vi "Teleop.vi"(10 "Match Info":T1={"Autonomous Elapsed Seconds"=0.0, "TeleOp Elapsed Seconds"=0.0, "Disabled Elapsed Seconds"=0.0, "Visited Autonomous"=FALSE, "Visited TeleOp"=FALSE, "Visited Disabled"=FALSE, "Autonomous Settings"={"Autonomous Style"=enum."Independent", "VI Refnum"=refnum}}, 11 "Call Context":T2) -> ()   [LabVIEW 2015]
doc: "This VI is called for each enabled TeleOp packet received from the DS. It is typically used to read from joysticks and other inputs and update I/O or setpoints for timed control loops. It should complete and return within 20 milliseconds or risk missing DS packets."
uses:
  <vilib>/Rock Robotics/WPI/DriverStation/WPI_DriverStationDerivedRobotMode.ctl
  <vilib>/Rock Robotics/WPI/DriverStation/WPI_DriverStationMatch Info.ctl
  Shooter/Implementation/Shooter Operations.ctl
  Support Code/Team900-VIs/Logitech/F510/F510-X.vi
  Shooter/Implementation/Shooter Published Globals.vi
  Drive/Implementation/Drive Operations.ctl
  Drive/Implementation/Drive Published Globals.vi
panel:
  in  "Angle":dbl=90.0 format="%#_13g"
  in  "Y":i32=40
  in  "X":i32=5
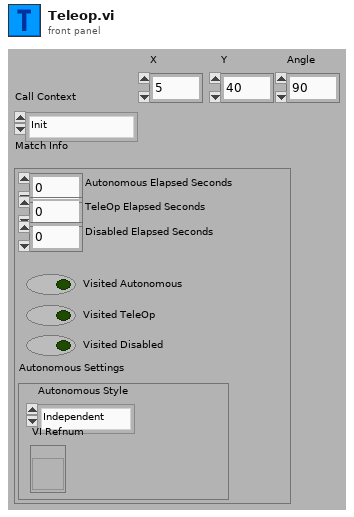
[diagram p1: front panel]
types:
  T1 = typedef "WPI_DriverStationMatch Info.ctl" = cluster{"Autonomous Elapsed Seconds":dbl, "TeleOp Elapsed Seconds":dbl, "Disabled Elapsed Seconds":dbl, "Visited Autonomous":bool, "Visited TeleOp":bool, "Visited Disabled":bool, "Autonomous Settings":cluster{"Autonomous Style":enum16{"Iterative", "Independent"}, "VI Refnum":refnum<vi>}}
  T2 = typedef "WPI_DriverStationDerivedRobotMode.ctl" = enum16{"Init", "Execute", "Stop"}
  T3 = typedef "Shooter Operations.ctl" = enum16{"Reserve", "Read Current", "Immediate", "Fire", "Aim"}
  T4 = typedef "Shooter Setpoints.ctl" = cluster{"Operation":T3, "Setpoint":dbl, "Duration":dbl}
  T5 = cluster{"A":bool, "B":bool, "X":bool, "Y":bool, "LB":bool, "RB":bool, "Back":bool, "Start":bool, "LC":bool, "RC":bool, "LT":bool, "RT":bool}
  T6 = typedef "Drive Operations.ctl" = enum16{"Reserve", "Read Current", "Immediate", "Turn to Angle", "Pick Up Ball", "Drive Straight", "Drive to Target (arc)"}
  T7 = typedef "Drive Setpoints.ctl" = cluster{"Operation":T6, "Left Setpoint":dbl, "Right Setpoint":dbl, "Duration":dbl, "Position":cluster{"X":dbl, "Y":dbl, "Angle":dbl, "Distance":dbl}, "Straight Setpoint":dbl}
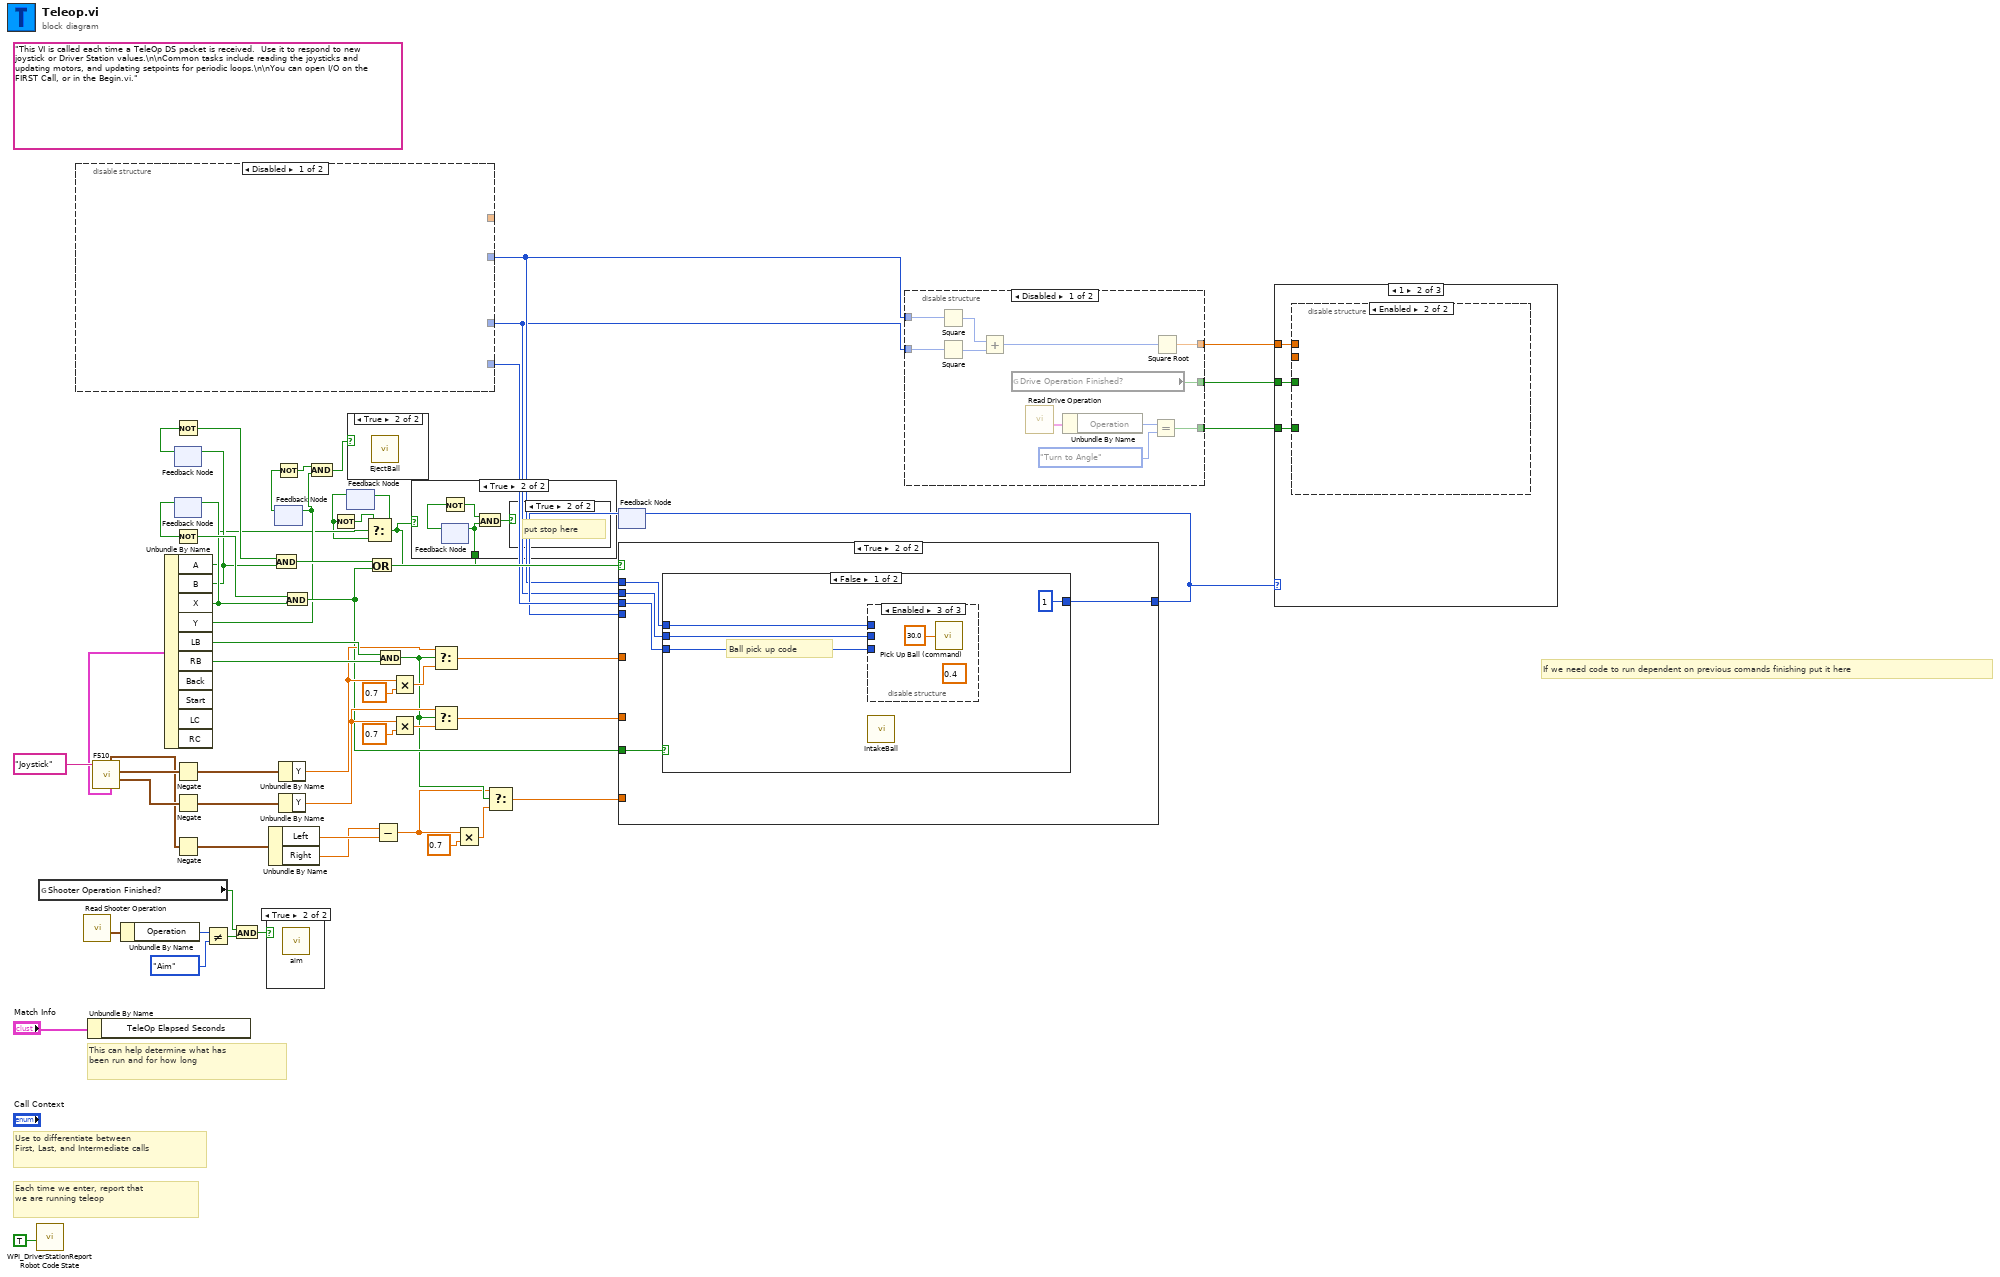
[diagram p0: block diagram]
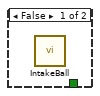
[diagram p2: hidden frame]
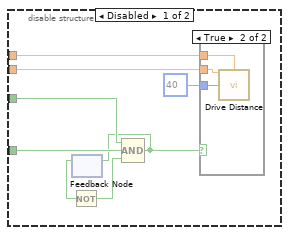
[diagram p8: hidden frame]
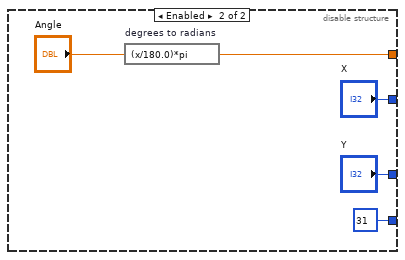
[diagram p11: hidden frame]
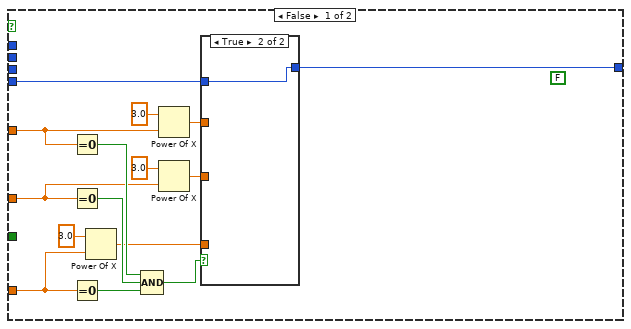
[diagram p12: hidden frame]
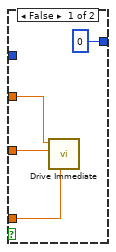
[diagram p13: hidden frame]
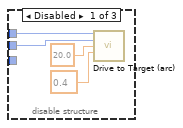
[diagram p14: hidden frame]
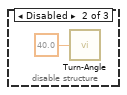
[diagram p15: hidden frame]
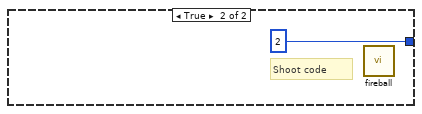
[diagram p16: hidden frame]
diagram:
  (unwired) "This VI is called each time a TeleOp DS packet is received.  Use it to respond to new joystick or Driver Station values.\n\nCommon tasks include reading the joysticks and updating motors, and updating setpoints for periodic loops.\n\nYou can open I/O on the FIRST Call, or in the Begin.vi."
  # "If we need code to run dependent on previous comands finishing put it here"
  # "Each time we enter, report that\nwe are running teleop"
  # "Use to differentiate between\nFirst, Last, and Intermediate calls"
  # "This can help determine what has\nbeen run and for how long"
  n1 = call <vilib>:"WPI_DriverStationReport Robot Code State.vi"("TeleOp"=TRUE ("Autonomous")) -> ()  [unwired: 10 in, 1 out]
  n2 = global read "Shooter Published Globals.vi" "Shooter Operation Finished?"() -> (w9:bool)
  n3 = disable-structure shown="Disabled" {
    disable-tunnel: [_ 31] -> w32
    disable-tunnel: [_ "Y"] -> w20
    disable-tunnel: [_ "X"] -> w21
    disable-tunnel: [_ w59] -> _
    frame Disabled {
    }
    frame Enabled {
      n4 = expression code="(x/180.0)*pi" "degrees to radians"("Angle") -> (w59:dbl)
    }
  }
  n5 = call "Read Shooter Operation.vi"() -> ("SubSystem Data"=w14:T4)  [unwired: 10 in, 1 out]
  n6 = Unbundle By Name("Match Info") -> ()  [unwired: 1 out]
  n7 = call-poly "F510.vi"("refnum name"="Joystick") -> ("Right Stick"=w54:cluster{"X":dbl, "Y":dbl}, "Left Stick"=w55:cluster{"X":dbl, "Y":dbl}, "Buttons"=w53:T5, "Triggers"=w52:cluster{"Left":dbl, "Right":dbl})  [unwired: 4 in, 3 out]
  n8 = Unbundle By Name(w14) -> ("Operation"=w13:T3)
  n9 = Unbundle By Name(w53) -> ("A"=w4:bool, "B"=w37:bool, "X"=w44:bool, "Y"=w6:bool, "LB"=w50:bool, "RB"=w51:bool)  [unwired: 4 out]
  n10 = feedback #1() -> (w36:bool)  [unwired: 1 in]
  n11 = Not(x=w36) -> (.not. x?=w38:bool)
  n12 = feedback-in #1(w37) -> ()
  n13 = feedback #2() -> (w41:bool)  [unwired: 1 in]
  n14 = feedback-in #2(w44) -> ()
  n15 = Not(x=w41) -> (.not. x?=w45:bool)
  n16 = Negate(x=w55) -> (-x=w16:cluster{"X":dbl, "Y":dbl})
  n17 = Negate(x=w54) -> (-x=w15:cluster{"X":dbl, "Y":dbl})
  n18 = Negate(x=w52) -> (-x=w17:cluster{"Left":dbl, "Right":dbl})
  n19 = Not Equal?(x=w13, y=Shooter_Operations."Aim") -> (x != y?=w11:bool)
  n20 = And(x=w9, y=w11) -> (x .and. y?=w10:bool)
  n21 = case shown="True" w10 {
    frame False {
    }
    frame True {
      n22 = call "aim.vi"() -> ()  [unwired: 11 in, 1 out]
    }
  }
  n23 = Unbundle By Name(w17) -> ("Left"=w27:dbl, "Right"=w26:dbl)
  n24 = And(x=w38, y=w37) -> (x .and. y?=w35:bool)
  n25 = feedback #3() -> (w8:bool)  [unwired: 1 in]
  n26 = Not(x=w8) -> (.not. x?=w7:bool)
  n27 = feedback-in #3(w6) -> ()
  n28 = Unbundle By Name(w16) -> ("Y"=w42:dbl)
  n29 = Unbundle By Name(w15) -> ("Y"=w43:dbl)
  n30 = And(x=w45, y=w44) -> (x .and. y?=w33:bool)
  n31 = And(x=w7, y=w6) -> (x .and. y?=w5:bool)
  n32 = feedback #4() -> (w2:bool)  [unwired: 1 in]
  n33 = Not(x=w2) -> (.not. x?=w3:bool)
  n34 = case shown="True" w5 {
    frame False {
    }
    frame True {
      n35 = call "EjectBall.vi"() -> ()  [unwired: 11 in, 1 out]
    }
  }
  n36 = Select(t=w3, s=w4, f=w2) -> (s? t:f=w1:bool)
  n37 = feedback-in #4(w1) -> ()
  n38 = Or(x=w35, y=w33) -> (x .or. y?=w34:bool)
  n39 = Subtract(x=w26, y=w27) -> (x-y=w25:dbl)
  n40 = And(x=w50, y=w51) -> (x .and. y?=w31:bool)
  n41 = Multiply(x=w42, y=0.7) -> (x*y=w47:dbl)
  n42 = Multiply(x=w43, y=0.7) -> (x*y=w49:dbl)
  n43 = case shown="True" w1 {
    tunnel: w1 -> [_ w65]
    frame False {
      n44 = call "IntakeBall.vi"() -> ()  [unwired: 11 in, 1 out]
    }
    frame True {
      n45 = feedback #5() -> (w67:bool)  [unwired: 1 in]
      n46 = Not(x=w67) -> (.not. x?=w66:bool)
      n47 = feedback-in #5(w65) -> ()
      n48 = And(x=w66, y=w65) -> (x .and. y?=w64:bool)
      n49 = case shown="True" w64 {
        frame False {
        }
        frame True {
          # "put stop here"
        }
      }
    }
  }
  n50 = Select(t=w42, s=w31, f=w47) -> (s? t:f=w40:dbl)
  n51 = Select(t=w43, s=w31, f=w49) -> (s? t:f=w39:dbl)
  n52 = Multiply(x=w25, y=0.7) -> (x*y=w29:dbl)
  n53 = Select(t=w25, s=w31, f=w29) -> (s? t:f=w28:dbl)
  n54 = feedback #6() -> (w23:i32)  [unwired: 1 in]
  n55 = case shown="True" w34 {
    tunnel: w40 -> [w78 _]
    tunnel: w39 -> [w73 _]
    tunnel: w33 -> [_ w92]
    tunnel: w32 -> [_ w91]
    tunnel: w20 -> [_ w90]
    tunnel: w21 -> [_ w89]
    tunnel: w28 -> [w71 _]
    tunnel: [w68 w88] -> w24
    tunnel: w23 -> [w69 _]
    frame False {
      (unwired) FALSE
      n56 = Equal To 0?(x=w78) -> (x = 0?=w81:bool)
      n57 = Equal To 0?(x=w73) -> (x = 0?=w82:bool)
      n58 = Equal To 0?(x=w71) -> (x = 0?=w79:bool)
      n59 = Power Of X(1:w71, 2:3.0 ("y")) -> (0:w70:dbl)
      n60 = Compound Arithmetic op=AND(w81, w82, w79) -> (w80:bool)
      n61 = Power Of X(1:w78, 2:3.0 ("y")) -> (0:w77:dbl)
      n62 = Power Of X(1:w73, 2:3.0 ("y")) -> (0:w74:dbl)
      n63 = case shown="True" w80 {
        tunnel: w77 -> [w86 _]
        tunnel: w74 -> [w85 _]
        tunnel: w70 -> [w84 _]
        tunnel: w69 -> [_ w87]
        tunnel: [0 w87] -> w68
        frame False {
          n64 = call "Drive Immediate.vi"("Straight Setpoint"=w84, "Right Setpoint"=w85, "Left Setpoint"=w86) -> ()  [unwired: 8 in, 1 out]
        }
        frame True {
        }
      }
    }
    frame True {
      n65 = case shown="False" w92 {
        tunnel: w91 -> [w96 _]
        tunnel: w90 -> [w94 _]
        tunnel: w89 -> [w95 _]
        tunnel: [1 2] -> w88
        frame False {
          # "Ball pick up code"
          n66 = disable-structure shown="Enabled" {
            disable-tunnel: w96 -> [_ _ _]
            disable-tunnel: w94 -> [w98 _ _]
            disable-tunnel: w95 -> [w100 _ _]
            frame Disabled {
              n67 = call "Drive to Target (arc).vi"("X"=w100, "Y"=w98, "Max time"=20.0, "Speed Setpoint (-1 to 1"=0.4) -> ()  [unwired: 10 in, 2 out]
            }
            frame Disabled {
              n68 = call "Turn-Angle.vi"("Max time"=40.0) -> ("Angle"=w102:dbl)  [unwired: 12 in, 2 out]
            }
            frame Enabled {
              (unwired) 0.4
              n69 = call "Pick Up Ball (command).vi"("Max time"=30.0) -> ()  [unwired: 13 in, 2 out]
            }
          }
          n70 = call "IntakeBall.vi"() -> ()  [unwired: 11 in, 1 out]
        }
        frame True {
          # "Shoot code"
          n71 = call "fireball.vi"() -> ()  [unwired: 11 in, 1 out]
        }
      }
    }
  }
  n72 = feedback-in #6(w24) -> ()
  n73 = disable-structure shown="Disabled" {
    disable-tunnel: [w115 _] -> w22
    disable-tunnel: w21 -> [w111 _]
    disable-tunnel: w20 -> [w110 _]
    disable-tunnel: [w109 _] -> w19
    disable-tunnel: [w105 _] -> w18
    frame Disabled {
      n74 = Square(x=w111) -> (x^2=w114:i32)
      n75 = Square(x=w110) -> (x^2=w112:i32)
      n76 = Add(x=w114, y=w112) -> (x+y=w113:i32)
      n77 = global read "Drive Published Globals.vi" "Drive Operation Finished?"() -> (w115:bool)
      n78 = call "Read Drive Operation.vi"() -> ("SubSystem Data"=w108:T7)  [unwired: 10 in, 1 out]
      n79 = Unbundle By Name(w108) -> ("Operation"=w107:T6)
      n80 = Equal?(x=w107, y=Drive_Operations."Turn to Angle") -> (x = y?=w105:bool)
      n81 = Square Root(x=w113) -> (sqrt(x)=w109:dbl)
    }
    frame Enabled {
    }
  }
  n82 = case shown="1" w24 {
    tunnel: w22 -> [_ w117 _]
    tunnel: w19 -> [_ w118 _]
    tunnel: w18 -> [_ w116 _]
    frame 0, Default {
    }
    frame 1 {
      n83 = disable-structure shown="Enabled" {
        disable-tunnel: _ -> [w126 _]
        disable-tunnel: w118 -> [w125 _]
        disable-tunnel: w117 -> [w124 _]
        disable-tunnel: w116 -> [w123 _]
        frame Disabled {
          n84 = feedback #7() -> (w121:bool)  [unwired: 1 in]
          n85 = Not(x=w121) -> (.not. x?=w120:bool)
          n86 = Compound Arithmetic op=AND(w124, w123, w120) -> (w122:bool)
          n87 = feedback-in #7(w122) -> ()
          n88 = case shown="True" w122 {
            tunnel: w126 -> [_ w129]
            tunnel: 40 -> [_ w128]
            tunnel: w125 -> [_ w127]
            frame False {
            }
            frame True {
              n89 = call "Drive Distance.vi"("Speed (-1 to 1)"=w129, "Distance (in)"=w127, "Max time"=w128) -> ()  [unwired: 11 in, 2 out]
            }
          }
        }
        frame Enabled {
        }
      }
    }
    frame 2 {
    }
  }
